vi "Write wrapnum.vi"(8 "error in (no error)":errorcluster, 10 "wrapnum":T1, 11 "CableWrapCommands in":refnum<class "CableWrapCommands.lvclass">) -> (0 "error out":errorcluster, 3 "CableWrapCommands out":refnum<class "CableWrapCommands.lvclass">)   [LabVIEW 2022 SP3, in "TCSDataDefinitions.lvlib" / "TCSCommand.lvlib" / "CableWrapCommands.lvlib" / "CableWrapCommands.lvclass"]
uses:
  CableWrapCommands.lvclass
  Enumerations/WrapnumTypes.ctl
  CableWrapCommands.lvclass/CableWrapCommands.ctl
  CableWrapCommands.lvlib
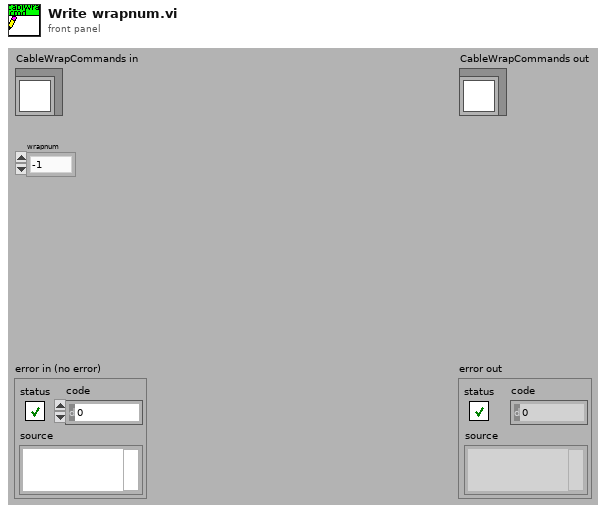
[diagram p1: front panel]
types:
  T1 = typedef "TCSDataDefinitions.lvlib/TCSCommand.lvlib/CableWrapCommands.lvlib/WrapnumTypes.ctl" = enum16{"-1", "0", "1"}
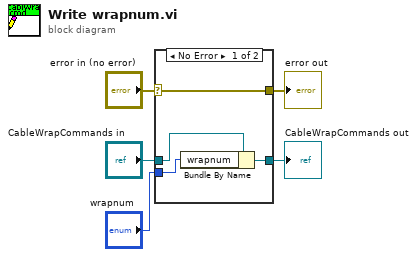
[diagram p0: block diagram]
diagram:
  n1 = case shown="No Error" "error in (no error)" {
    selector: "error in (no error)" -> [w9 w10]
    tunnel: [w9 w10] -> w4
    tunnel: [w7 w11] -> w2
    tunnel: "CableWrapCommands in" -> [w8 w11]
    tunnel: "wrapnum" -> [w6 _]
    frame No Error {
      n2 = Bundle By Name(cluster=w8, "wrapnum"=w6) -> (w7:refnum<class "CableWrapCommands.lvclass">)
    }
    frame Error {
    }
  }
  "error out" <- w4
  "CableWrapCommands out" <- w2
